vi "InitAnalogSettings.vi"(1 "error in (no error)":errorcluster) -> (0 "error out":errorcluster)   [LabVIEW 2009]
uses:
  AnalogSettings.ctt
  <vilib>/Utility/config.llb/NI_LVConfig.lvlib
panel:
  out "file created?":bool
  in  "Analog Settings":T1={"PCI 671x Device Number"=1, "Samples per Unit"=10}
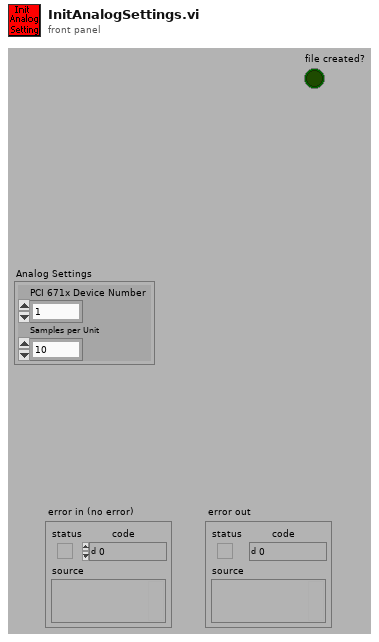
[diagram p1: front panel]
types:
  T1 = typedef "AnalogSettings.ctt" = cluster{"PCI 671x Device Number":u32, "Samples per Unit":u32}
  T2 = typedef "NI_LVConfig.lvlib/Config Data RefNum.ctl" = refnum<k1>
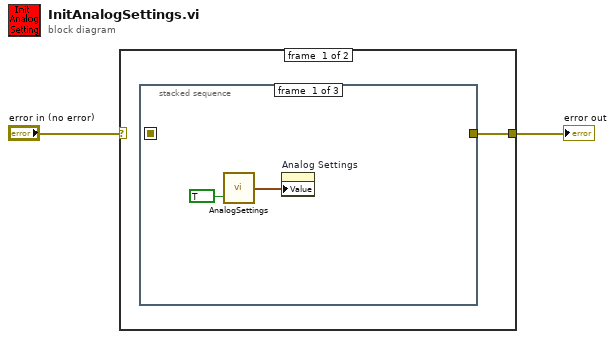
[diagram p0: block diagram]
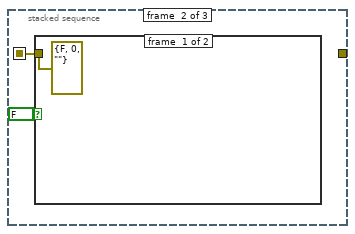
[diagram p2: hidden frame]
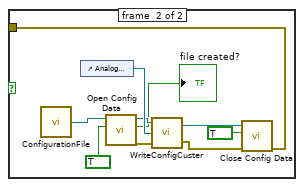
[diagram p3: hidden frame]
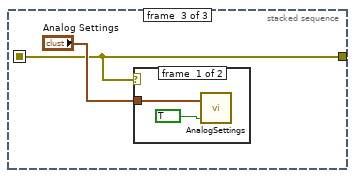
[diagram p4: hidden frame]
diagram:
  n1 = case shown="No Error" "error in (no error)" {
    selector: "error in (no error)" -> [_ w23]
    tunnel: [w3 w23] -> w1
    frame #0 {
      n2 = stacked-sequence {
        seq-local: [_ w7 _] -> [_ _ w19]
        tunnel: [_ _ w19] -> w3
        frame #0 {
          n3 = call "AnalogSettings.vi"("Get/Set"=TRUE) -> ("Analog Settings (output)"=w4:T1)  [unwired: 1 in]
          n4 = property on="Analog Settings" class="Clust (strict)"("Value"=w4) -> ()  [unwired: 2 in, 2 out]
        }
        frame #1 {
          n5 = case shown="True" FALSE {
            tunnel: [errorcluster {"status"=FALSE, "code"=0, "source"=""} ("error out") w17] -> w7
            frame #0 {
            }
            frame #1 {
              n6 = call "ConfigurationFile.vi"() -> ("Configuration File (output)"=w12:path)  [unwired: 2 in]
              n7 = control-ref of="Analog Settings"() -> (w14:refnum<vi>)
              n8 = call <vilib>:"Open Config Data.vi"("create file if necessary (T)"=TRUE ("create file if necessary? (T)"), "configuration file path"=w12) -> ("error out"=w10:errorcluster, "file created?"=→"file created?":bool, "refnum"=w11:T2)  [unwired: 7 in]
              n9 = call "WriteConfigCuster.vi"("error in (no error)"=w10, "Ctrl Reference"=w14, "ConfigFile (input)"=w11) -> ("error out"=w15:errorcluster, "ConfigFile (output)"=w16:T2)
              n10 = call "Close Config Data.vi"("error in (no error)"=w15, "write configuration file? (T)"=TRUE ("write configuration file? (F)"), "refnum"=w16) -> ("error out"=w17:errorcluster)  [unwired: 8 in]
            }
          }
        }
        frame #2 {
          n11 = case shown="No Error" w19 {
            tunnel: "Analog Settings" -> [w22 _]
            frame #0 {
              n12 = call "AnalogSettings.vi"("Get/Set"=TRUE ("Set"), "Analog Settings (input)"=w22) -> ()  [unwired: 1 out]
            }
            frame #1 {
            }
          }
        }
      }
    }
    frame #1 {
    }
  }
  "error out" <- w1
